vi "TCP Read Stream.vi"(5 "file dialog info":T1={"prompt"="Please select a file to write to", "pattern"="*", "default name"=""}, 6 "chunk size (4096)":i32=4096, 7 "binary":bool, 8 "error in (no error)":errorcluster, 9 "header (\"\")":string, 10 "data file (<NAP>)":path=path "", 11 "connection":refnum<k5>) -> (0 "error out":errorcluster, 1 "data":string, 2 "data file out":path, 3 "duplicate connection":refnum<k5>, 4 "file error":errorcluster)   [LabVIEW 2017, in "NI_FTP.lvlib"]
doc: "Read data from a TCP connection until the connection is closed.\n\"header\" is written in front of the data read.\nIf \"data file\" is specified, the data is written to a new \"data file\", otherwise it is returned in \"data\".\nIf \"binary\" is FALSE, EOLN characters in the data will be converted to the system EOLN characters (when written to file) or '\\n' when returned in data.\n\"chunk size\" determines how many bytes at a time are read from the file"
uses:
  <vilib>/FTP/NI_FTP.lvlib
panel:
  in  "Num Retries":i32=250
  in  "(no error)":errorcluster
  in  "refnum":refnum<file>
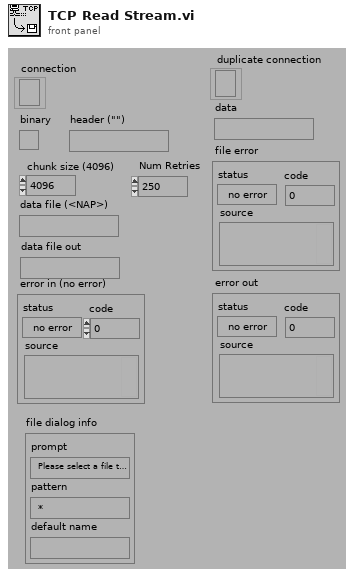
[diagram p1: front panel]
types:
  T1 = cluster{"prompt":string, "pattern":string, "default name":string}
  T2 = enum16{"open", "replace", "create", "open or create", "replace or create", "replace or create with confirmation"}
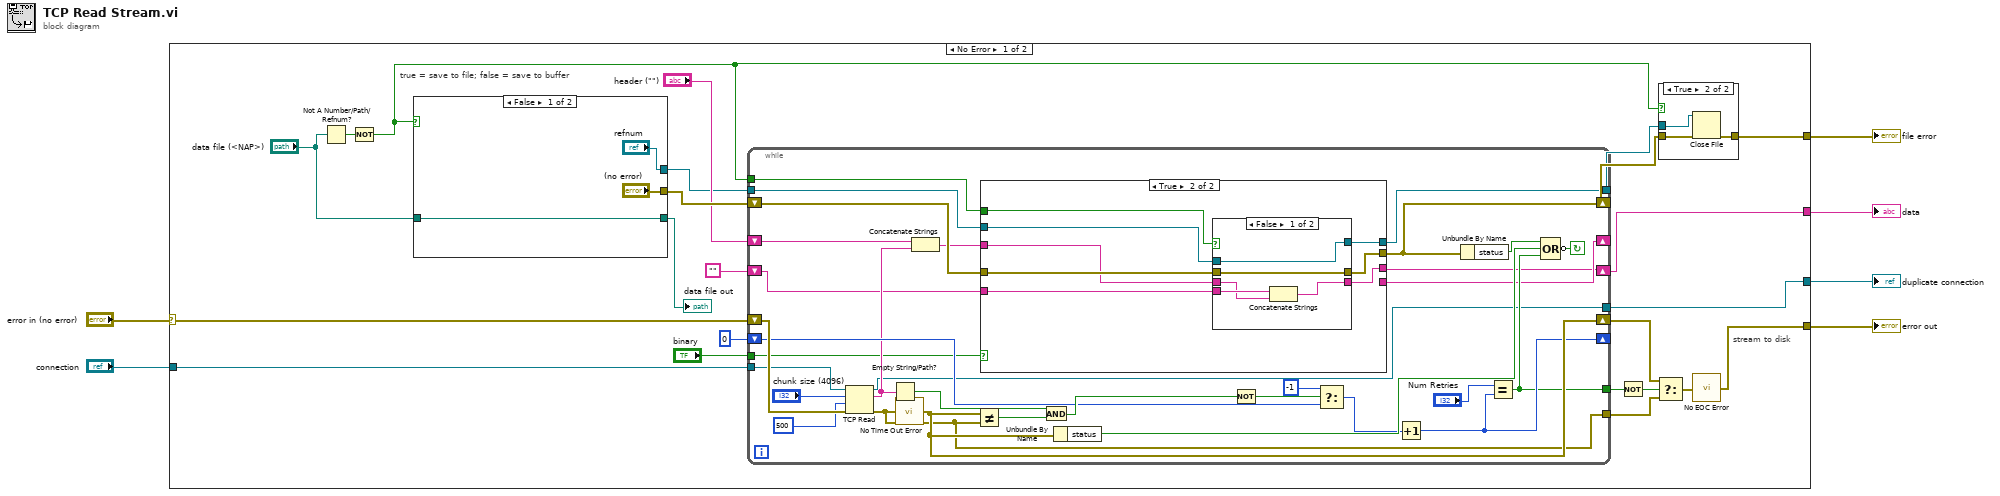
[diagram p0: block diagram]
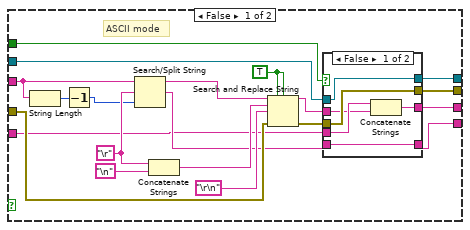
[diagram p2: hidden frame]
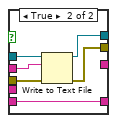
[diagram p3: hidden frame]
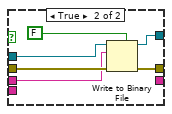
[diagram p4: hidden frame]
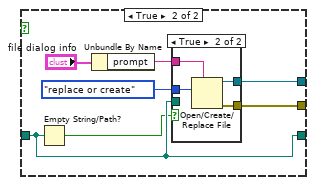
[diagram p6: hidden frame]
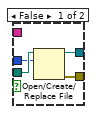
[diagram p7: hidden frame]
diagram:
  n1 = case shown="No Error" "error in (no error)" {
    selector: "error in (no error)" -> [w12 w135]
    tunnel: [w26 w135] -> w6
    tunnel: [w25 w136] -> w5
    tunnel: [w23 _] -> w4
    tunnel: [w7 _] -> w3
    tunnel: "connection" -> [w13 w136]
    frame No Error {
      # "true = save to file; false = save to buffer"
      # "stream to disk"
      n2 = Not A Number/Path/Refnum?(number/path/refnum="data file (<NAP>)") -> (NaN/Path/Refnum?=w27:bool)
      n3 = Not(x=w27) -> (.not. x?=w20:bool)
      n4 = case shown="False" w20 {
        tunnel: "data file (<NAP>)" -> [w117 w123]
        tunnel: ["refnum" w124] -> w10
        tunnel: ["(no error)" w125] -> w28
        tunnel: [w117 w123] -> w21
        frame False {
        }
        frame True {
          n5 = Empty String/Path?(string/path=w123) -> (empty?=w122:bool)
          n6 = Unbundle By Name("file dialog info") -> ("prompt"=w120:string)
          n7 = case shown="True" w122 {
            tunnel: T2."replace or create" ("operation (0:open)") -> [w127 w134]
            tunnel: [w130 w133] -> w125
            tunnel: [w129 w132] -> w124
            tunnel: w123 -> [w128 _]
            tunnel: w120 -> [_ w131]
            frame False {
              n8 = Open/Create/Replace File(file path (use dialog)=w128, operation (0:open)=w127) -> (refnum out=w129:refnum<file>, error out=w130:errorcluster)  [unwired: 4 in, 1 out]
            }
            frame True {
              n9 = Open/Create/Replace File(prompt=w131, operation (0:open)=w134) -> (refnum out=w132:refnum<file>, error out=w133:errorcluster)  [unwired: 4 in, 1 out]
            }
          }
        }
      }
      "data file out" <- w21
      n10 = while {
        tunnel: [w32] -> w25
        tunnel: w13 -> [w59]
        tunnel: w20 -> [w35]
        shift-left: "header (\"\")" -> [w40]
        shift-right: [w37] -> _
        shift-left: w12 -> [w61]
        shift-right: [w53] -> w15
        shift-left: w28 -> [w60]
        shift-right: [w36] -> w24
        shift-right: [w44] -> _
        shift-left: 0 -> [w47]
        tunnel: [w43] -> w17
        tunnel: [w42] -> w16
        tunnel: "binary" -> [w38]
        tunnel: w10 -> [w34]
        tunnel: [w33] -> w9
        shift-right: [w30] -> w7
        shift-left: "" -> [w31]
        stop <- w55 continue-if-true
        n11 = TCP Read(connection ID=w59, bytes to read="chunk size (4096)", error in (no error)=w61, 9:500 ("timeout ms (25000)")) -> (connection ID out=w32:refnum<k5>, data out=w41:string, error out=w42:errorcluster)  [unwired: 1 out]
        n12 = Empty String/Path?(string/path=w41) -> (empty?=w52:bool)
        n13 = call <vilib>:"No Time Out Error.vi"("error in (no error)"=w42) -> ("error out"=w53:errorcluster)  [unwired: 14 out]
        n14 = Concatenate Strings(w40, w41) -> (w39:string)
        n15 = Not Equal?(x=w53, y=w42) -> (x != y?=w51:bool)
        n16 = case shown="True" w38 {
          tunnel: w39 -> [w66 w98]
          tunnel: w60 -> [w77 w99]
          tunnel: [w70 _] -> w37
          tunnel: [w74 w97] -> w36
          tunnel: w35 -> [w76 w101]
          tunnel: w34 -> [w73 w100]
          tunnel: [w71 w96] -> w33
          tunnel: [w63 w95] -> w30
          tunnel: w31 -> [w62 w94]
          frame False {
            w78 = TRUE ("replace all? (F)")
            w68 = "\r"
            # "ASCII mode"
            n17 = String Length(string=w66) -> (length=w69:i32)
            n18 = Decrement(x=w69) -> (x-1=w67:i32)
            n19 = Search/Split String(string=w66, search string/char (-)=w68, offset (0)=w67) -> (substring before match=w65:string, match + rest of string=w64:string)  [unwired: 1 out]
            n20 = Concatenate Strings(w68, "\n") -> (w80:string)
            n21 = Search and Replace String(replace all?=w78, case sensitive?=w78, input string=w65, search string=w80, replace string="\r\n", error in=w77) -> (result string=w72:string, error out=w75:errorcluster)  [unwired: 4 out]
            n22 = case shown="False" w76 {
              tunnel: w75 -> [w87 w93]
              tunnel: [w87 w92] -> w74
              tunnel: w73 -> [w86 w91]
              tunnel: w72 -> [w83 w90]
              tunnel: [w86 w89] -> w71
              tunnel: [w85 w88] -> w70
              tunnel: w64 -> [w85 w88]
              tunnel: [w82 _] -> w63
              tunnel: w62 -> [w84 _]
              frame False {
                n23 = Concatenate Strings(w84, w83) -> (w82:string)
              }
              frame True {
                n24 = Write to Text File(file (use dialog)=w91, text=w90, error in=w93) -> (refnum out=w89:refnum<file>, error out=w92:errorcluster)  [unwired: 2 out]
              }
            }
          }
          frame True {
            n25 = case shown="False" w101 {
              tunnel: w100 -> [w106 w112]
              tunnel: w99 -> [w105 w111]
              tunnel: w98 -> [w103 w110]
              tunnel: [w105 w109] -> w97
              tunnel: [w106 w108] -> w96
              tunnel: [w102 _] -> w95
              tunnel: w94 -> [w104 _]
              frame False {
                n26 = Concatenate Strings(w104, w103) -> (w102:string)
              }
              frame True {
                n27 = Write to Binary File(file (use dialog)=w112, data=w110, error in=w111, 5:FALSE ("prepend array or string size? (T)")) -> (refnum out=w108:refnum<file>, error out=w109:errorcluster)  [unwired: 3 out]
              }
            }
          }
        }
        n28 = And(x=w52, y=w51) -> (x .and. y?=w50:bool)
        n29 = Unbundle By Name(w53) -> ("status"=w56:bool)
        n30 = Not(x=w50) -> (.not. x?=w49:bool)
        n31 = Select(t=-1, s=w49, f=w47) -> (s? t:f=w46:i32)
        n32 = Increment(x=w46) -> (x+1=w44:i32)
        n33 = Unbundle By Name(w36) -> ("status"=w57:bool)
        n34 = Equal?(x="Num Retries", y=w44) -> (x = y?=w43:bool)
        n35 = Compound Arithmetic op=OR(w57, w56, w43) -> (invert w55:bool)
      }
      n36 = Not(x=w17) -> (.not. x?=w18:bool)
      n37 = Select(t=w15, s=w18, f=w16) -> (s? t:f=w14:errorcluster)
      n38 = case shown="True" w20 {
        tunnel: w24 -> [w113 w116]
        tunnel: [w113 w115] -> w23
        tunnel: w9 -> [_ w114]
        frame False {
        }
        frame True {
          n39 = Close File(refnum=w114, error in=w116) -> (error out=w115:errorcluster)  [unwired: 1 out]
        }
      }
      n40 = call <vilib>:"No EOC Error.vi"("error in (no error)"=w14) -> ("error out"=w26:errorcluster)  [unwired: 4 out]
    }
    frame Error {
    }
  }
  "data" <- w3
  "error out" <- w6
  "duplicate connection" <- w5
  "file error" <- w4
